vi "Compute Fit Curve v4.vi"(0 "X Array in":dbl[](array[numeric]), 1 "# Points":u32, 2 "Use Same Number of Points as Histogram":bool, 5 "Best Fit in":dbl[](array[numeric]), 7 "Y Array in":dbl[](array[numeric]), 9 "Fit Settings":T1={"Use Original Plot # Points"=TRUE, "# Fit Plot Points"=0, "Fit Method"=0, "Weighted Fit"=FALSE, "Show All Fit Components"=FALSE, "Axis Type"=0, "Show Fit Residuals"=FALSE, "Residual Type"=enum."Standard"} {"Axis Type" items=["Linear", "Logarithmic"]; "Fit Method" items=["Least Square", "Least Absolute Residual", "Bisquare"]}, 11 "Error In":errorcluster, 12 "Fit Model":T5, 13 "Fit Parameters":variant, 14 "Ramp Type":T3 items=["Linear", "Logarithmic"]) -> (3 "Array of Plots (Fit, Components, Residuals)":cluster{"X Array":dbl[], "Y Array":dbl[]}[](array[cluster]), 4 "Fitted Plot":cluster{"X Array":dbl[], "Y Array":dbl[]}, 6 "Array of Component Plots":cluster{"X Array":dbl[], "Y Array":dbl[]}[](array[cluster]), 8 "Residual Plot":cluster{"X Array":dbl[], "Y Array":dbl[]}, 10 "Residual Type":string, 15 "Error Out":errorcluster)   [LabVIEW 2019]
uses:
  Fit Models.ctl
  Calc/Ramp Type.ctl
  Fit Settings.ctl
  <vilib>/Analysis/6fits.llb/Curve Fitting Criteria.ctl
  Residual Type.ctl
  Gaussian/Gaussian Fit Results v2.ctl
  Two Connected Gaussians/Two H-Connected Gaussians Fit Parameters.ctl
  Two Connected Asymmetric Gaussians/Two H-Connected Asymmetric Gaussians Fit Parameters.ctl
  Asymmetric Gaussian/Asymmetric Gaussian Fit Results v2.ctl
  Two Connected Asymmetric Gaussians/Two T-Connected Asymmetric Gaussians Fit Parameters.ctl
  Two Connected Gaussians/Two T-Connected Gaussians Fit Parameters.ctl
  Asymmetric Lorentzian/Asymmetric Lorentzian Fit Results v2.ctl
  Gaussian-Lorentzian/Gaussian-Lorentzian Fit Results v2.ctl
  Lorentzian-Gaussian/Lorentzian-Gaussian Fit Results v2.ctl
  Lorentzian/Lorentzian Fit Results v2.ctl
  Single Exponential/Single Exponential Fit Parameters v2.ctl
  Double Exponential/Double Exponential Fit Parameters v2.ctl
  ACF-CCF/2D ACF/2D Gaussian ACF Fit Results.ctl
  ACF-CCF/2D ACF/2D Gaussian + Blinking ACF Fit Results.ctl
  ACF-CCF/2D ACF/2D Gaussian + Flow ACF Fit Results.ctl
  ACF-CCF/3D ACF/3D Gaussian ACF Fit Results.ctl
  ACF-CCF/3D ACF/3D Gaussian + Blinking ACF Fit Results.ctl
  <vilib>/Analysis/NI_AALBase.lvlib
  <vilib>/Analysis/NI_AALPro.lvlib
panel:
  out "Array of Plots (Fit, Components, Residuals)":cluster{"X Array":dbl[], "Y Array":dbl[]}[](array[cluster])
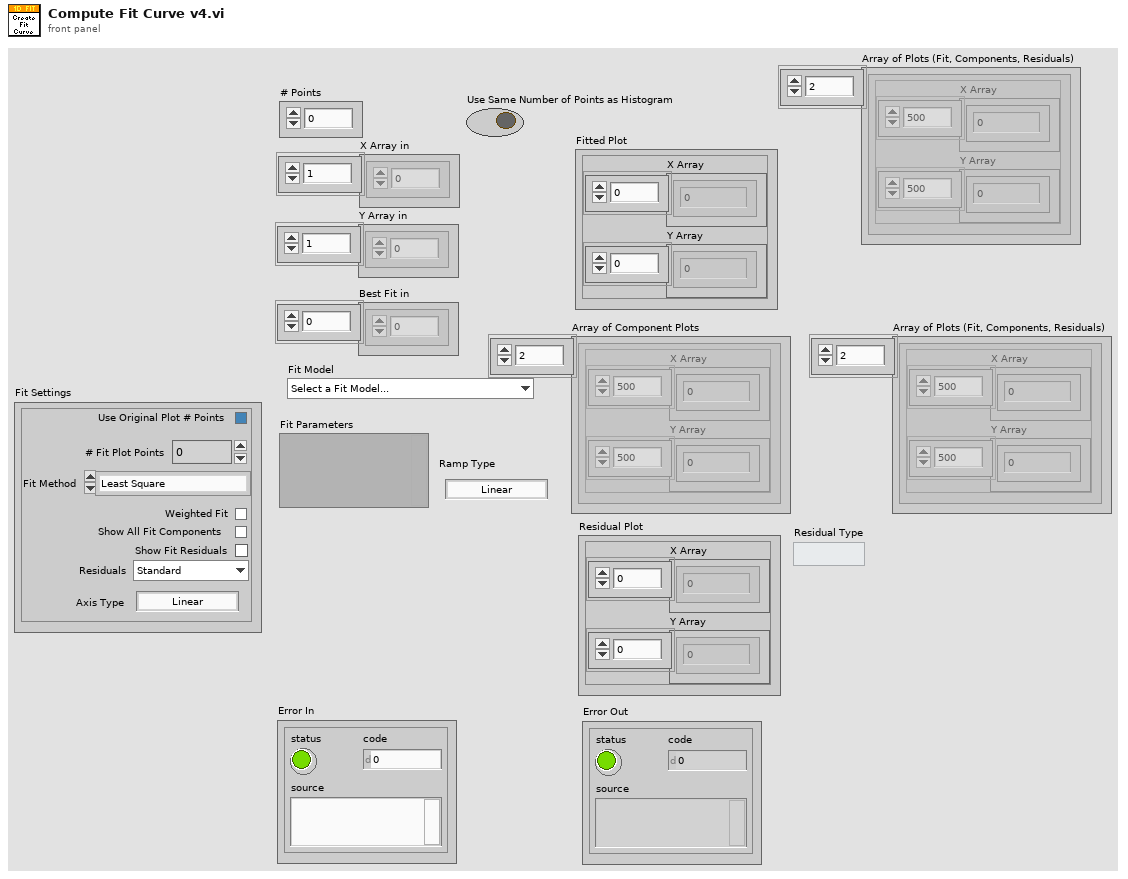
[diagram p1: front panel]
types:
  T1 = typedef "Fit Settings.ctl" = cluster{"Use Original Plot # Points":bool, "# Fit Plot Points":u32, "Fit Method":T2, "Weighted Fit":bool, "Show All Fit Components":bool, "Axis Type":T3, "Show Fit Residuals":bool, "Residual Type":T4}
  T2 = typedef "NI_AALPro.lvlib/Curve Fitting Criteria.ctl" = u16
  T3 = typedef "Ramp Type.ctl" = u16
  T4 = typedef "Residual Type.ctl" = enum16{"Standard", "Normalized", "Reduced"}
  T5 = typedef "Fit Models.ctl" = enum16{"Select a Fit Model...", "           Single Peak", "Gaussian", "Asymmetric Gaussian", "Lorentzian", "Asymmetric Lorentzian", "Gaussian/Lorentzian", "Lorentzian/Gaussian", "           Double Peak", "Two Gaussians", "Two Asymmetric Gaussians", "Two H-Connected Gaussians", "Two T-Connected Gaussians", "Two H-Connected Asymmetric Gaussians", "Two T-Connected Asymmetric Gaussians", "           Triple Peak", "Three Gaussians", "Three Asymmetric Gaussians", "              Decays", "1-Exponential", "IRF*PSED", "2-Exponentials", "               ACF", "2D Gaussian ACF", "2D Gaussian + Blinking ACF", "2D Gaussian + Flow ACF", "3D Gaussian ACF", "3D Gaussian + Blinking ACF", "             Multiplot", "2D Gaussian ACF & 2D Gaussian + Flow ACF"}
  T6 = typedef "Gaussian Fit Results v2.ctl" = cluster{"Amplitude":dbl, "Peak":dbl, "SDV":dbl, "FWHM":dbl, "Integral":dbl, "RMSE":dbl, "R^2":dbl}
  T7 = typedef "Two H-Connected Gaussians Fit Parameters.ctl" = cluster{"Gaussian Parameters":T6[], "Bridge Amplitude ":dbl}
  T8 = typedef "Two H-Connected Asymmetric Gaussians Fit Parameters.ctl" = cluster{"Asymmetric Gaussian Parameters":T9[], "Bridge Amplitude":dbl}
  T9 = typedef "Asymmetric Gaussian Fit Results v2.ctl" = cluster{"Amplitude":dbl, "Peak":dbl, "SDV-":dbl, "SDV+":dbl, "Mean":dbl, "SDV":dbl, "FWHM":dbl, "Integral":dbl, "RMSE":dbl, "R^2":dbl}
  T10 = typedef "Two T-Connected Asymmetric Gaussians Fit Parameters.ctl" = cluster{"Asymmetric Gaussian Parameters":T9[], "Bridge Amplitude":dbl, "Bridge Slope":dbl}
  T11 = typedef "Two T-Connected Gaussians Fit Parameters.ctl" = cluster{"Gaussian Parameters":T6[], "Bridge Amplitude ":dbl, "Bridge Slope":dbl}
  T12 = typedef "Asymmetric Lorentzian Fit Results v2.ctl" = cluster{"Amplitude":dbl, "Peak":dbl, "FWHM-":dbl, "FWHM+":dbl, "Integral":dbl, "RMSE":dbl, "R^2":dbl}
  T13 = typedef "Gaussian-Lorentzian Fit Results v2.ctl" = cluster{"Amplitude":dbl, "Peak":dbl, "SDV-":dbl, "FWHM+":dbl, "Mean":dbl, "FWHM":dbl, "Integral":dbl, " RMSE":dbl, "R^2":dbl}
  T14 = typedef "Lorentzian-Gaussian Fit Results v2.ctl" = cluster{"Amplitude":dbl, "Peak":dbl, "FWHM-":dbl, "SDV+":dbl, "Mean":dbl, "FWHM":dbl, "Integral":dbl, "RMSE":dbl, "R^2":dbl}
  T15 = typedef "Lorentzian Fit Results v2.ctl" = cluster{"Amplitude":dbl, "Peak":dbl, "FWHM":dbl, "Integral":dbl, "RMSE":dbl, "R^2":dbl}
  T16 = typedef "Single Exponential Fit Parameters v2.ctl" = cluster{"Amplitude":dbl, "Time Constant":dbl, "Baseline":dbl, "Mean":dbl, "SDV":dbl, "FWHM":dbl, "Integral":dbl, "MSE":dbl, "R^2":dbl}
  T17 = typedef "Double Exponential Fit Parameters v2.ctl" = cluster{"A1":dbl, "tau1":dbl, "A2":dbl, "tau2":dbl, "Baseline":dbl, "Mean":dbl, "SDV":dbl, "Integral":dbl, "MSE":dbl, "R^2":dbl}
  T18 = typedef "2D Gaussian ACF Fit Results.ctl" = cluster{"Amplitude":dbl, "Diffusion Time":dbl, "RMSE":dbl, "R^2":dbl}
  T19 = typedef "2D Gaussian + Blinking ACF Fit Results.ctl" = cluster{"Amplitude":dbl, "Diffusion Time":dbl, "Blinking Fraction":dbl, "Blinking Time Constant":dbl, "RMSE":dbl, "R^2":dbl}
  T20 = typedef "2D Gaussian + Flow ACF Fit Results.ctl" = cluster{"Amplitude":dbl, "Diffusion Time":dbl, "Translation Time":dbl, "RMSE":dbl, "R^2":dbl}
  T21 = typedef "3D Gaussian ACF Fit Results.ctl" = cluster{"Amplitude":dbl, "Diffusion Time":dbl, "Aspect Ratio":dbl, "RMSE":dbl, "R^2":dbl}
  T22 = typedef "3D Gaussian + Blinking ACF Fit Results.ctl" = cluster{"Amplitude":dbl, "Diffusion Time":dbl, "Aspect Ratio":dbl, "Blinking Fraction":dbl, "Blinking Time Constant":dbl, "RMSE":dbl, "R^2":dbl}
  T23 = typedef "IRF(X)PSED Fit Parameters.ctl" = cluster{"Offset":dbl, "Amplitudes":dbl[], "Time Constants":dbl[], "Baseline":dbl, "Lifetime":dbl, "IRF order":dbl, "Period":dbl, "SDV":dbl, "FWHM":dbl, "Integral":dbl, "MSE":dbl, "R^2":dbl}
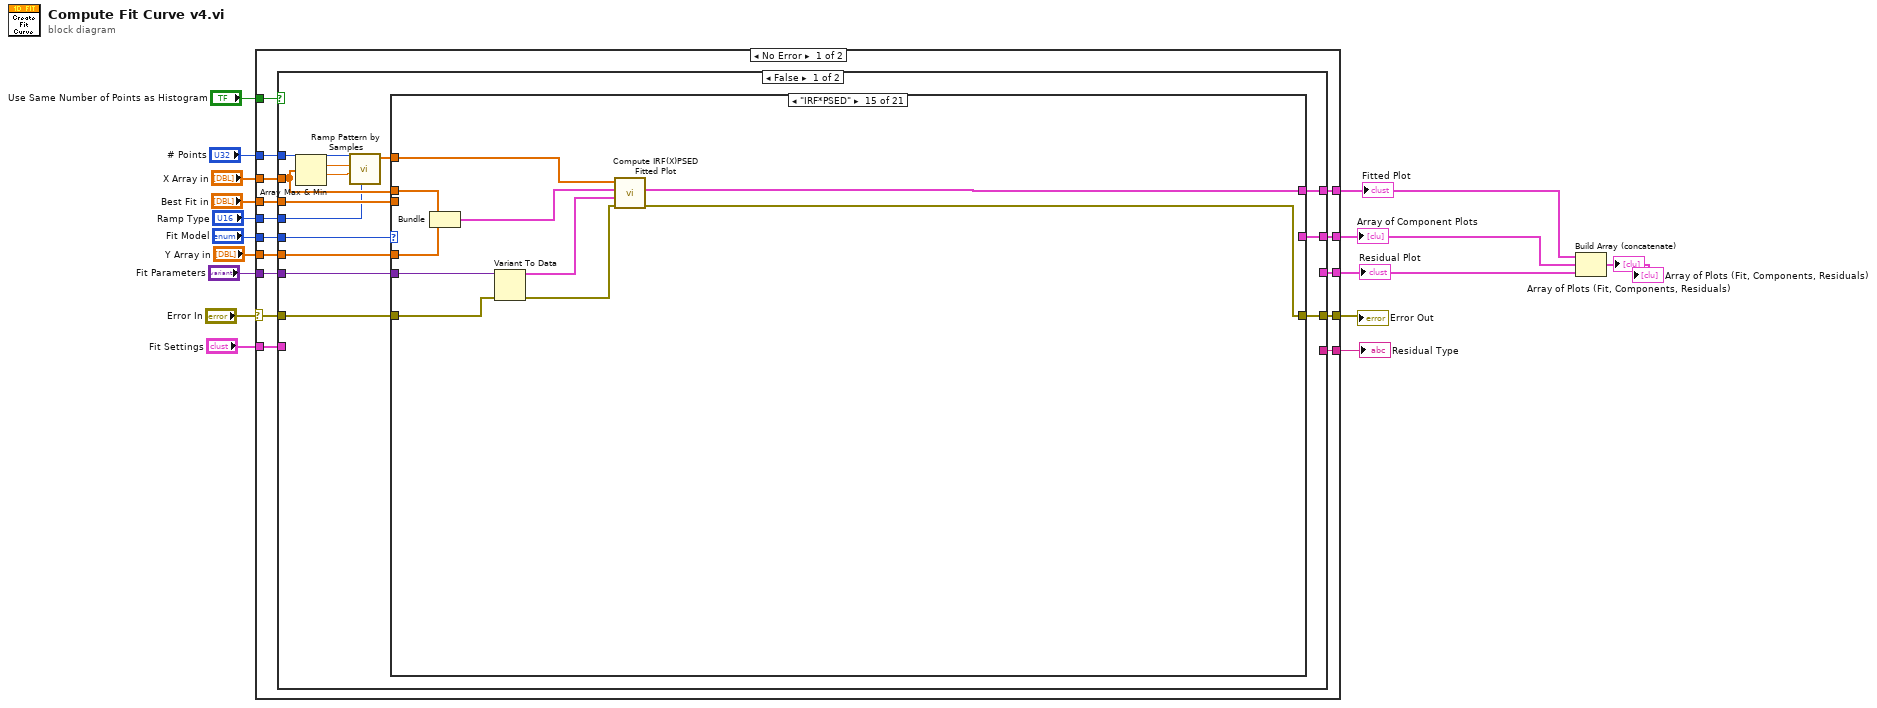
[diagram p0: block diagram]
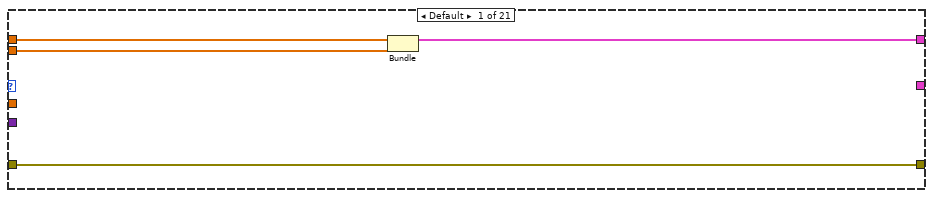
[diagram p2: hidden frame]
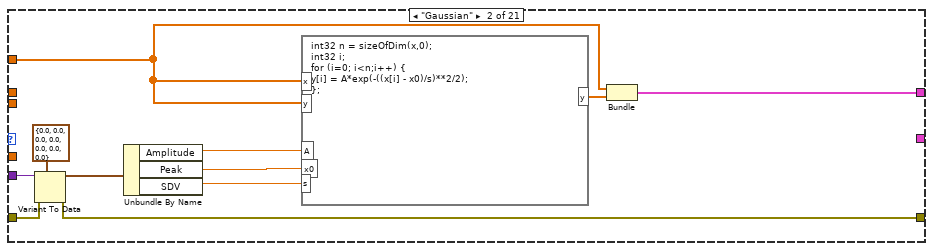
[diagram p3: hidden frame]
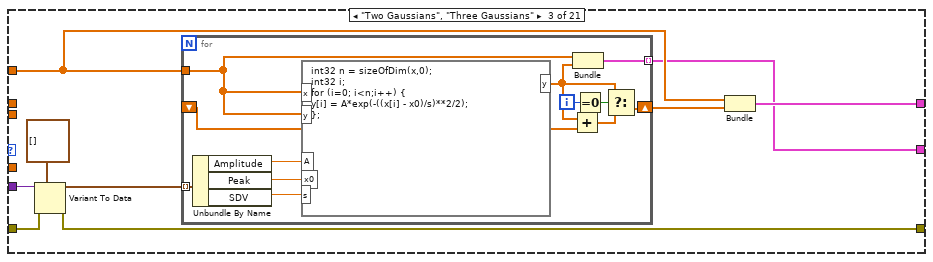
[diagram p4: hidden frame]
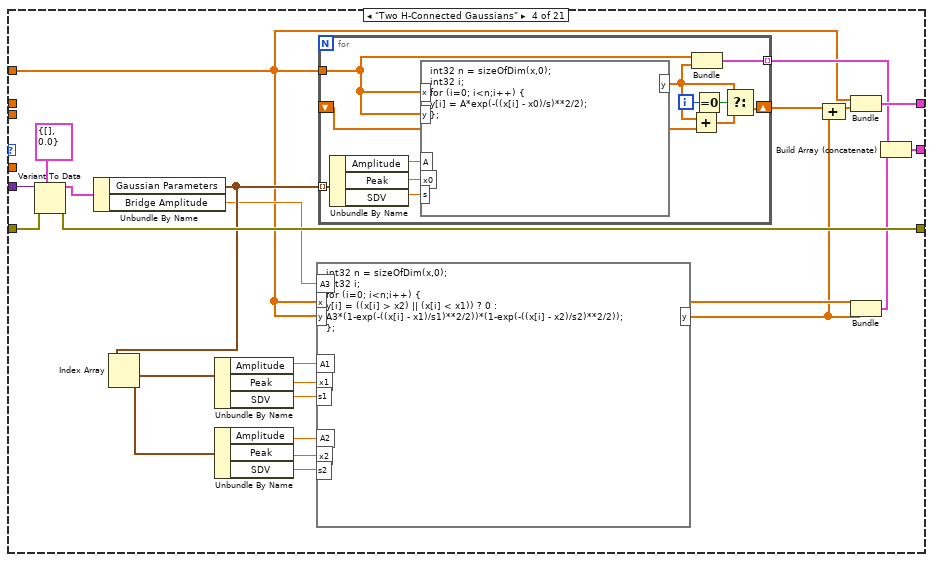
[diagram p5: hidden frame]
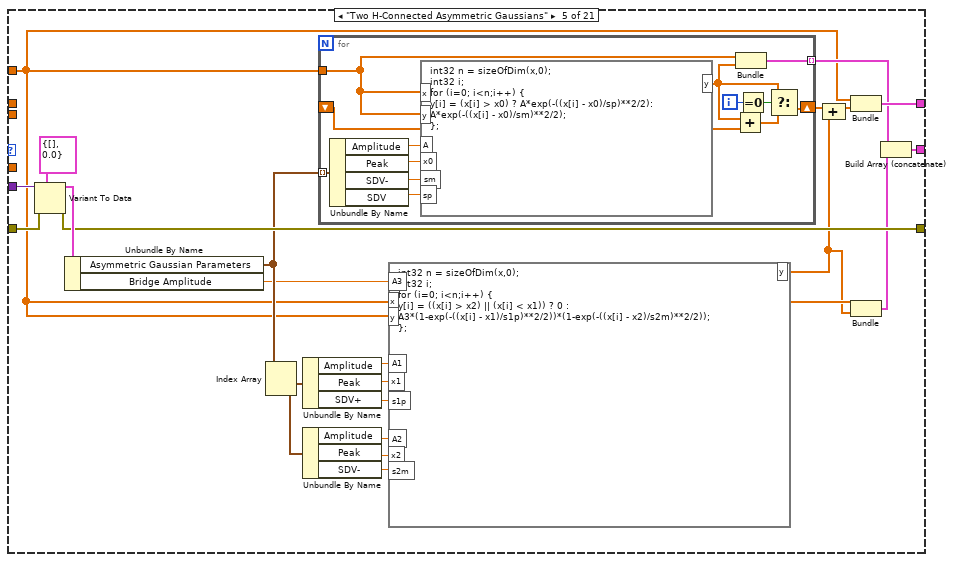
[diagram p6: hidden frame]
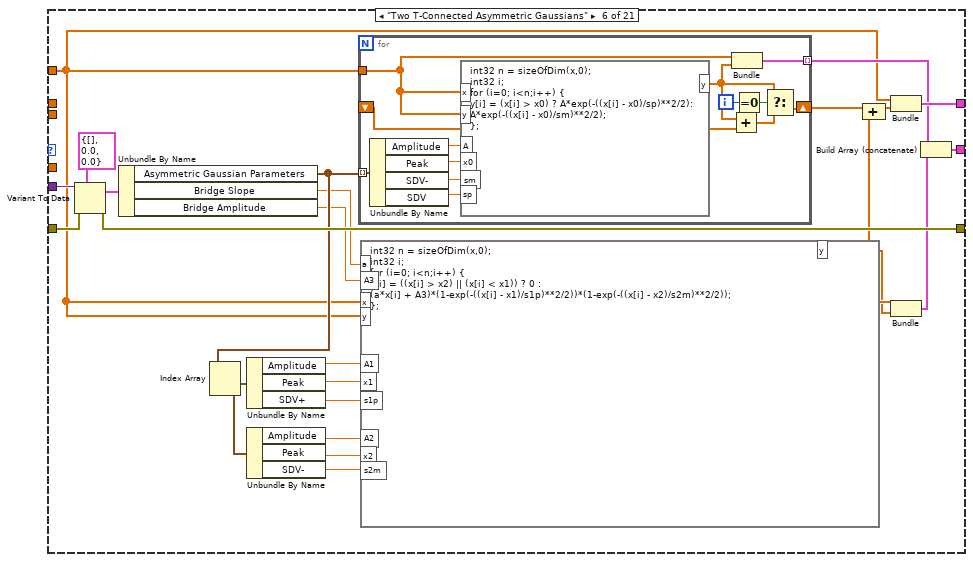
[diagram p7: hidden frame]
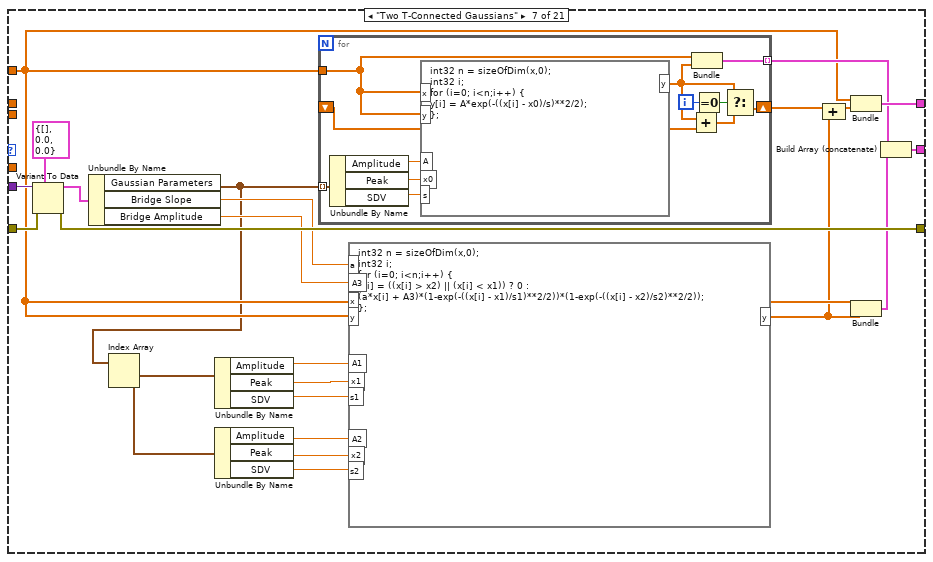
[diagram p8: hidden frame]
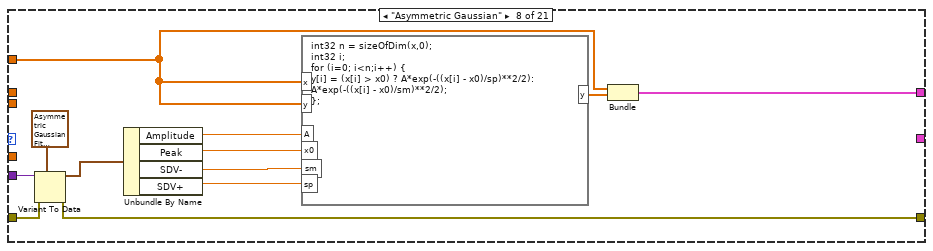
[diagram p9: hidden frame]
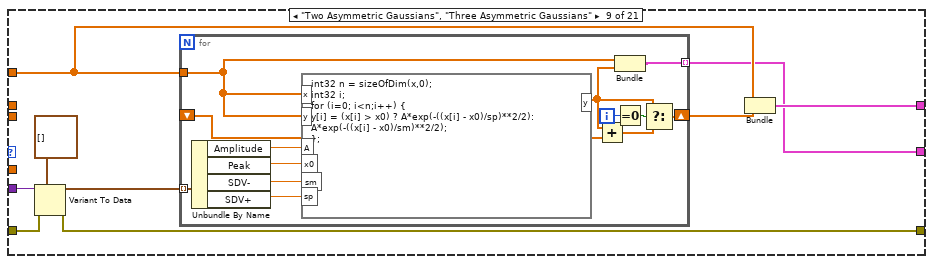
[diagram p10: hidden frame]
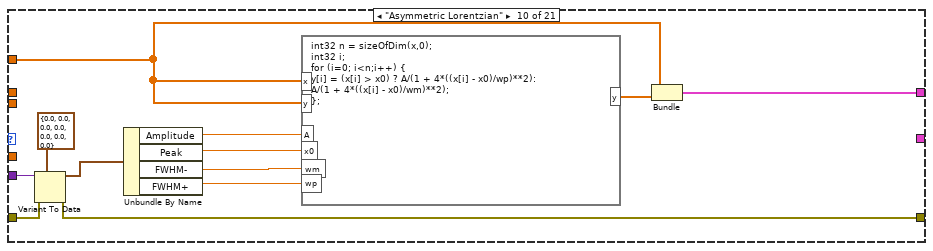
[diagram p11: hidden frame]
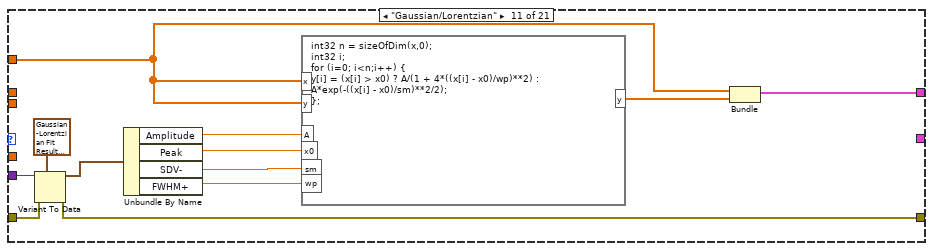
[diagram p12: hidden frame]
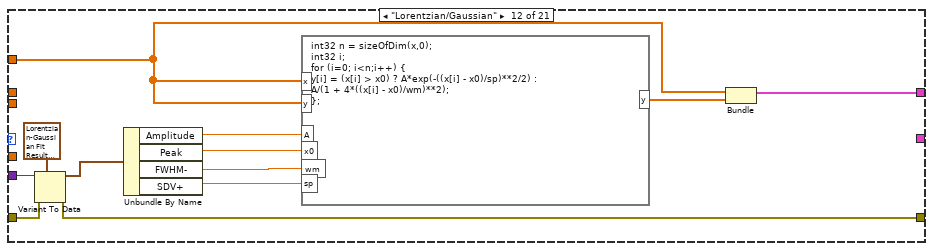
[diagram p13: hidden frame]
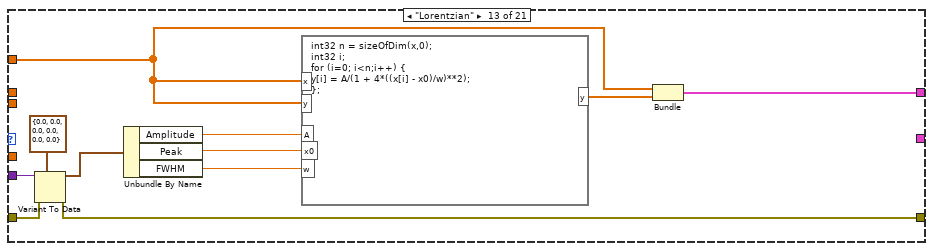
[diagram p14: hidden frame]
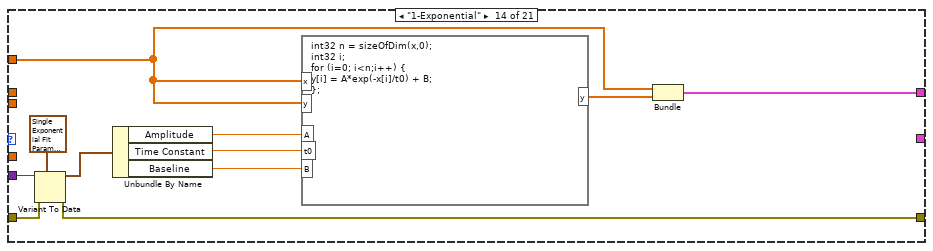
[diagram p15: hidden frame]
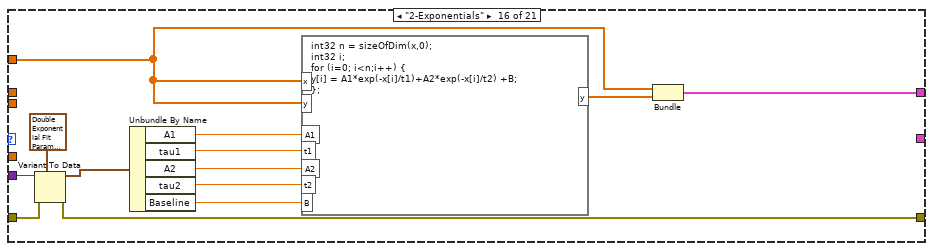
[diagram p16: hidden frame]
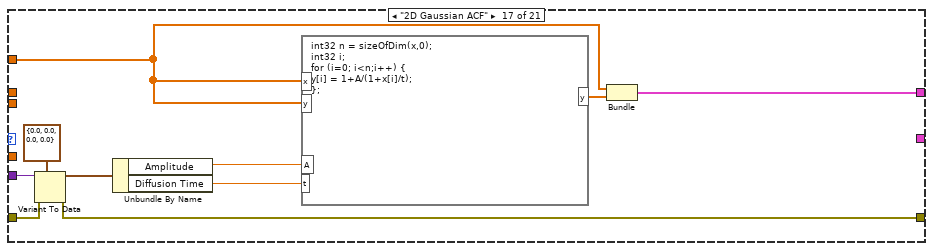
[diagram p17: hidden frame]
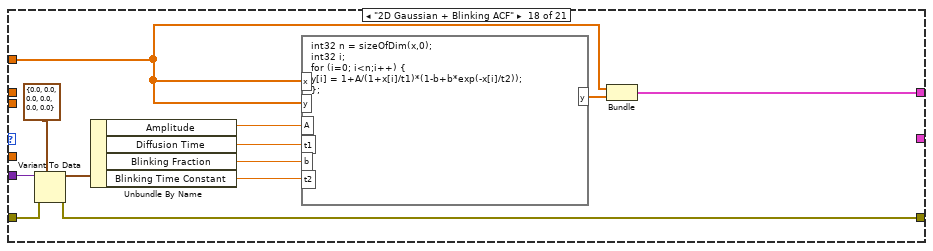
[diagram p18: hidden frame]
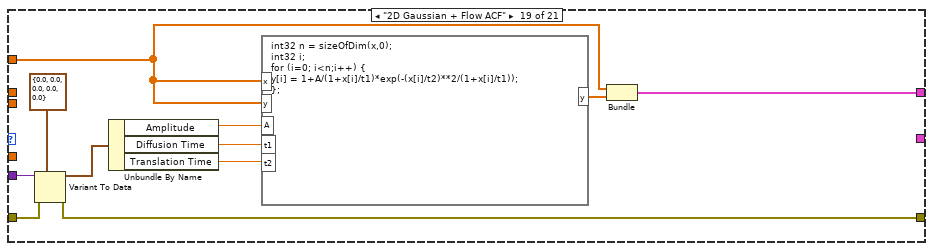
[diagram p19: hidden frame]
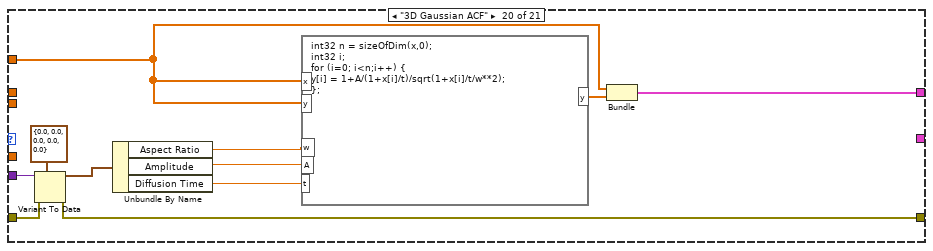
[diagram p20: hidden frame]
diagram:
  n1 = case shown="No Error" "Error In" {
    selector: "Error In" -> [w25 w434]
    tunnel: "Fit Model" -> [w31 _]
    tunnel: [w24 w434] -> w14
    tunnel: "Use Same Number of Points as Histogram" -> [w30 _]
    tunnel: "X Array in" -> [w29 w433]
    tunnel: "Best Fit in" -> [w28 w432]
    tunnel: "# Points" -> [w27 _]
    tunnel: "Fit Parameters" -> [w26 _]
    tunnel: [w22 _] -> w3
    tunnel: [w23 w431] -> w2
    tunnel: "Ramp Type" -> [w21 _]
    tunnel: [w20 _] -> w4
    tunnel: "Y Array in" -> [w19 _]
    tunnel: "Fit Settings" -> [w18 _]
    tunnel: [w17 _] -> w5
    frame No Error {
      n2 = case shown="False" w30 {
        tunnel: w31 -> [w45 _]
        tunnel: w29 -> [w38 w409]
        tunnel: w28 -> [w37 w406]
        tunnel: w27 -> [w44 _]
        tunnel: w26 -> [w40 _]
        tunnel: w25 -> [w39 w411]
        tunnel: [w36 w411] -> w24
        tunnel: [w35 w410] -> w23
        tunnel: [w34 _] -> w22
        tunnel: w21 -> [w33 _]
        tunnel: [_ w408] -> w20
        tunnel: w19 -> [w32 w407]
        tunnel: w18 -> [_ w402]
        tunnel: [_ w398] -> w17
        frame False {
          n3 = Array Max & Min(array=w38) -> (max value=w43:dbl, min value=w42:dbl)  [unwired: 2 out]
          n4 = call <vilib>:"Ramp Pattern by Samples.vi"("type"=w33, "start"=w42, "end"=w43, "samples"=w44) -> ("Ramp Pattern"=w41:dbl[])  [unwired: 6 in, 1 out]
          n5 = case shown="\"IRF*PSED\"" w45 {
            tunnel: w41 -> [_ w50 w63 w86 w122 w159 w196 w227 w240 w261 w273 w284 w296 w309 w326 w332 w341 w354 w365 w375 w389]
            tunnel: w40 -> [_ w60 w69 w104 w139 w176 w213 w237 w246 w271 w283 w295 w306 w317 w325 w340 w350 w362 w373 w384 w397]
            tunnel: w39 -> [w49 w58 w68 w103 w138 w175 w212 w236 w245 w270 w282 w294 w305 w316 w318 w339 w348 w361 w372 w382 w396]
            tunnel: w38 -> [w47 _ _ _ _ _ _ _ _ _ _ _ _ _ w324 _ _ _ _ _ _]
            tunnel: w37 -> [w48 _ _ _ _ _ _ _ _ _ _ _ _ _ _ _ _ _ _ _ _]
            tunnel: [w49 w53 w66 w101 w136 w173 w210 w230 w243 w264 w276 w288 w300 w312 w327 w335 w344 w357 w368 w378 w392] -> w36
            tunnel: [w46 w51 w62 w99 w134 w171 w208 w226 w239 w260 w272 w286 w298 w311 w321 w334 w342 w355 w366 w376 w390] -> w35
            tunnel: [_ _ w61 w93 w128 w165 w203 _ w238 _ _ _ _ _ _ _ _ _ _ _ _] -> w34
            tunnel: w32 -> [_ _ _ _ _ _ _ _ _ _ _ _ _ _ w323 _ _ _ _ _ _]
            frame Default {
              n6 = Bundle("X Array in"=w47, "Best Fit in"=w48) -> (w46:cluster{"X Array in":dbl[], "Best Fit in":dbl[]})  [unwired: 1 in]
            }
            frame "Gaussian" {
              n7 = Variant To Data(error in=w58, type=T6 {"Amplitude"=0.0, "Peak"=0.0, "SDV"=0.0, "FWHM"=0.0, "Integral"=0.0, "RMSE"=0.0, "R^2"=0.0} ("Gaussian Fit Parameters"), Variant=w60) -> (data=w57:T6, error out=w53:errorcluster)
              n8 = Unbundle By Name(w57) -> ("Amplitude"=w56:dbl, "Peak"=w55:dbl, "SDV"=w54:dbl)
              n9 = formula code="int32 n = sizeOfDim(x,0);\nint32 i;\nfor (i=0; i<n;i++) {\ny[i] = A*exp(-((x[i] - x0)/s)**2/2);\n};"("A"=w56, "x0"=w55, "s"=w54, "x"=w50, "y"=w50) -> ("y"=w52:dbl[])
              n10 = Bundle("Ramp Pattern"=w50, "y"=w52) -> (w51:cluster{"Ramp Pattern":dbl[], "y":dbl[]})  [unwired: 1 in]
            }
            frame "Two Gaussians", "Three Gaussians" {
              n11 = Variant To Data(error in=w68, type=T6[] [] ("Two Gaussians Fit Parameters"), Variant=w69) -> (data=w67:T6[], error out=w66:errorcluster)
              n12 = for {
                tunnel: w67 -> [w81] mode=indexing
                tunnel: w63 -> [w71]
                shift-right: [w74] -> w64
                shift-left: _ -> [w75]
                tunnel: [w70] -> w61 mode=indexing
                i -> [w77]
                n13 = Unbundle By Name(w81) -> ("Amplitude"=w80:dbl, "Peak"=w79:dbl, "SDV"=w78:dbl)
                n14 = formula code="int32 n = sizeOfDim(x,0);\nint32 i;\nfor (i=0; i<n;i++) {\ny[i] = A*exp(-((x[i] - x0)/s)**2/2);\n};"("A"=w80, "x0"=w79, "s"=w78, "x"=w71, "y"=w71) -> ("y"=w72:dbl[])
                n15 = Add(x=w72, y=w75) -> (x+y=w73:dbl[])
                n16 = Bundle("Ramp Pattern"=w71, "y"=w72) -> (w70:cluster{"Ramp Pattern":dbl[], "y":dbl[]})  [unwired: 1 in]
                n17 = Equal To 0?(x=w77) -> (x = 0?=w76:bool)
                n18 = Select(t=w72, s=w76, f=w73) -> (s? t:f=w74:dbl[])
              }
              n19 = Bundle("Ramp Pattern"=w63, "y"=w64) -> (w62:cluster{"Ramp Pattern":dbl[], "y":dbl[]})  [unwired: 1 in]
            }
            frame "Two H-Connected Gaussians" {
              n20 = Variant To Data(error in=w103, type=T7 {"Gaussian Parameters"=[], "Bridge Amplitude "=0.0} ("Bridged Gaussians Parameters"), Variant=w104) -> (data=w102:T7, error out=w101:errorcluster)
              n21 = Unbundle By Name(w102) -> ("Gaussian Parameters"=w97:T6[], "Bridge Amplitude"=w94:dbl)
              n22 = Index Array(array=w97) -> (element #1=w96:T6, element #2=w95:T6)  [unwired: 2 in]
              n23 = Unbundle By Name(w96) -> ("Amplitude"=w92:dbl, "Peak"=w91:dbl, "SDV"=w90:dbl)
              n24 = Unbundle By Name(w95) -> ("Amplitude"=w87:dbl, "Peak"=w88:dbl, "SDV"=w89:dbl)
              n25 = formula code="int32 n = sizeOfDim(x,0);\nint32 i;\nfor (i=0; i<n;i++) {\ny[i] = ((x[i] > x2) || (x[i] < x1)) ? 0 : \nA3*(1-exp(-((x[i] - x1)/s1)**2/2))*(1-exp(-((x[i] - x2)/s2)**2/2));\n};"("A1"=w92, "x1"=w91, "s1"=w90, "x"=w86, "y"=w86, "A2"=w87, "x2"=w88, "s2"=w89, "A3"=w94) -> ("y"=w83:dbl[])
              n26 = for {
                tunnel: w97 -> [w116] mode=indexing
                tunnel: w86 -> [w106]
                shift-right: [w109] -> w100
                shift-left: _ -> [w110]
                tunnel: [w105] -> w98 mode=indexing
                i -> [w112]
                n27 = Unbundle By Name(w116) -> ("Amplitude"=w115:dbl, "Peak"=w114:dbl, "SDV"=w113:dbl)
                n28 = formula code="int32 n = sizeOfDim(x,0);\nint32 i;\nfor (i=0; i<n;i++) {\ny[i] = A*exp(-((x[i] - x0)/s)**2/2);\n};"("A"=w115, "x0"=w114, "s"=w113, "x"=w106, "y"=w106) -> ("y"=w107:dbl[])
                n29 = Add(x=w107, y=w110) -> (x+y=w108:dbl[])
                n30 = Bundle("Ramp Pattern"=w106, "y"=w107) -> (w105:cluster{"Ramp Pattern":dbl[], "y":dbl[]})  [unwired: 1 in]
                n31 = Equal To 0?(x=w112) -> (x = 0?=w111:bool)
                n32 = Select(t=w107, s=w111, f=w108) -> (s? t:f=w109:dbl[])
              }
              n33 = Compound Arithmetic op=ADD(w100, w83) -> (w84:dbl[])
              n34 = Bundle("Ramp Pattern"=w86, w84) -> (w99:cluster{"Ramp Pattern":dbl[], dbl[]})  [unwired: 1 in]
              n35 = Bundle("Ramp Pattern"=w86, "y"=w83) -> (w85:cluster{"Ramp Pattern":dbl[], "y":dbl[]})  [unwired: 1 in]
              n36 = Build Array (concatenate)(w98, w85) -> (w93:cluster{"Ramp Pattern":dbl[], "y":dbl[]}[])
            }
            frame "Two H-Connected Asymmetric Gaussians" {
              n37 = Variant To Data(error in=w138, type=T8 {"Asymmetric Gaussian Parameters"=[], "Bridge Amplitude"=0.0} ("output cluster"), Variant=w139) -> (data=w137:T8, error out=w136:errorcluster)
              n38 = Unbundle By Name(w137) -> ("Asymmetric Gaussian Parameters"=w132:T9[], "Bridge Amplitude"=w129:dbl)
              n39 = Index Array(array=w132) -> (element #1=w131:T9, element #2=w130:T9)  [unwired: 2 in]
              n40 = Unbundle By Name(w131) -> ("Amplitude"=w127:dbl, "Peak"=w126:dbl, "SDV+"=w118:dbl)
              n41 = Unbundle By Name(w130) -> ("Amplitude"=w123:dbl, "Peak"=w124:dbl, "SDV-"=w125:dbl)
              n42 = for {
                tunnel: w132 -> [w152] mode=indexing
                tunnel: w122 -> [w141]
                shift-right: [w144] -> w135
                shift-left: _ -> [w145]
                tunnel: [w140] -> w133 mode=indexing
                i -> [w147]
                n43 = Unbundle By Name(w152) -> ("Amplitude"=w151:dbl, "Peak"=w150:dbl, "SDV-"=w149:dbl, "SDV"=w148:dbl)
                n44 = formula code="int32 n = sizeOfDim(x,0);\nint32 i;\nfor (i=0; i<n;i++) {\ny[i] = (x[i] > x0) ? A*exp(-((x[i] - x0)/sp)**2/2):\nA*exp(-((x[i] - x0)/sm)**2/2);\n};"("A"=w151, "x0"=w150, "sm"=w149, "sp"=w148, "x"=w141, "y"=w141) -> ("y"=w142:dbl[])
                n45 = Add(x=w142, y=w145) -> (x+y=w143:dbl[])
                n46 = Bundle("Ramp Pattern"=w141, "y"=w142) -> (w140:cluster{"Ramp Pattern":dbl[], "y":dbl[]})  [unwired: 1 in]
                n47 = Equal To 0?(x=w147) -> (x = 0?=w146:bool)
                n48 = Select(t=w142, s=w146, f=w143) -> (s? t:f=w144:dbl[])
              }
              n49 = formula code="int32 n = sizeOfDim(x,0);\nint32 i;\nfor (i=0; i<n;i++) {\ny[i] = ((x[i] > x2) || (x[i] < x1)) ? 0 : \nA3*(1-exp(-((x[i] - x1)/s1p)**2/2))*(1-exp(-((x[i] - x2)/s2m)**2/2));\n};"("A1"=w127, "x1"=w126, "x"=w122, "y"=w122, "A2"=w123, "x2"=w124, "s2m"=w125, "A3"=w129, "s1p"=w118) -> ("y"=w119:dbl[])
              n50 = Compound Arithmetic op=ADD(w135, w119) -> (w120:dbl[])
              n51 = Bundle("Ramp Pattern"=w122, w120) -> (w134:cluster{"Ramp Pattern":dbl[], dbl[]})  [unwired: 1 in]
              n52 = Bundle("Ramp Pattern"=w122, "y"=w119) -> (w121:cluster{"Ramp Pattern":dbl[], "y":dbl[]})  [unwired: 1 in]
              n53 = Build Array (concatenate)(w133, w121) -> (w128:cluster{"Ramp Pattern":dbl[], "y":dbl[]}[])
            }
            frame "Two T-Connected Asymmetric Gaussians" {
              n54 = Variant To Data(error in=w175, type=T10 {"Asymmetric Gaussian Parameters"=[], "Bridge Amplitude"=0.0, "Bridge Slope"=0.0} ("Two T-Connected Asymmetric Gaussian Parameters"), Variant=w176) -> (data=w174:T10, error out=w173:errorcluster)
              n55 = Unbundle By Name(w174) -> ("Asymmetric Gaussian Parameters"=w169:T9[], "Bridge Slope"=w166:dbl, "Bridge Amplitude"=w154:dbl)
              n56 = Index Array(array=w169) -> (element #1=w168:T9, element #2=w167:T9)  [unwired: 2 in]
              n57 = Unbundle By Name(w168) -> ("Amplitude"=w164:dbl, "Peak"=w163:dbl, "SDV+"=w155:dbl)
              n58 = Unbundle By Name(w167) -> ("Amplitude"=w160:dbl, "Peak"=w161:dbl, "SDV-"=w162:dbl)
              n59 = for {
                tunnel: w169 -> [w189] mode=indexing
                tunnel: w159 -> [w178]
                shift-right: [w181] -> w172
                shift-left: _ -> [w182]
                tunnel: [w177] -> w170 mode=indexing
                i -> [w184]
                n60 = Unbundle By Name(w189) -> ("Amplitude"=w188:dbl, "Peak"=w187:dbl, "SDV-"=w186:dbl, "SDV"=w185:dbl)
                n61 = formula code="int32 n = sizeOfDim(x,0);\nint32 i;\nfor (i=0; i<n;i++) {\ny[i] = (x[i] > x0) ? A*exp(-((x[i] - x0)/sp)**2/2):\nA*exp(-((x[i] - x0)/sm)**2/2);\n};"("A"=w188, "x0"=w187, "sm"=w186, "sp"=w185, "x"=w178, "y"=w178) -> ("y"=w179:dbl[])
                n62 = Add(x=w179, y=w182) -> (x+y=w180:dbl[])
                n63 = Bundle("Ramp Pattern"=w178, "y"=w179) -> (w177:cluster{"Ramp Pattern":dbl[], "y":dbl[]})  [unwired: 1 in]
                n64 = Equal To 0?(x=w184) -> (x = 0?=w183:bool)
                n65 = Select(t=w179, s=w183, f=w180) -> (s? t:f=w181:dbl[])
              }
              n66 = formula code="int32 n = sizeOfDim(x,0);\nint32 i;\nfor (i=0; i<n;i++) {\ny[i] = ((x[i] > x2) || (x[i] < x1)) ? 0 : \n(a*x[i] + A3)*(1-exp(-((x[i] - x1)/s1p)**2/2))*(1-exp(-((x[i] - x2)/s2m)**2/2));\n};"("A1"=w164, "x1"=w163, "x"=w159, "y"=w159, "A2"=w160, "x2"=w161, "s2m"=w162, "a"=w166, "s1p"=w155, "A3"=w154) -> ("y"=w156:dbl[])
              n67 = Compound Arithmetic op=ADD(w172, w156) -> (w157:dbl[])
              n68 = Bundle("Ramp Pattern"=w159, w157) -> (w171:cluster{"Ramp Pattern":dbl[], dbl[]})  [unwired: 1 in]
              n69 = Bundle("Ramp Pattern"=w159, "y"=w156) -> (w158:cluster{"Ramp Pattern":dbl[], "y":dbl[]})  [unwired: 1 in]
              n70 = Build Array (concatenate)(w170, w158) -> (w165:cluster{"Ramp Pattern":dbl[], "y":dbl[]}[])
            }
            frame "Two T-Connected Gaussians" {
              n71 = Variant To Data(error in=w212, type=T11 {"Gaussian Parameters"=[], "Bridge Amplitude "=0.0, "Bridge Slope"=0.0} ("Bridged Gaussians Parameters"), Variant=w213) -> (data=w211:T11, error out=w210:errorcluster)
              n72 = Unbundle By Name(w211) -> ("Gaussian Parameters"=w190:T6[], "Bridge Slope"=w204:dbl, "Bridge Amplitude"=w192:dbl)
              n73 = Index Array(array=w190) -> (element #1=w206:T6, element #2=w205:T6)  [unwired: 2 in]
              n74 = Unbundle By Name(w206) -> ("Amplitude"=w202:dbl, "Peak"=w201:dbl, "SDV"=w200:dbl)
              n75 = Unbundle By Name(w205) -> ("Amplitude"=w197:dbl, "Peak"=w198:dbl, "SDV"=w199:dbl)
              n76 = for {
                tunnel: w190 -> [w225] mode=indexing
                tunnel: w196 -> [w215]
                shift-right: [w218] -> w209
                shift-left: _ -> [w219]
                tunnel: [w214] -> w207 mode=indexing
                i -> [w221]
                n77 = Unbundle By Name(w225) -> ("Amplitude"=w224:dbl, "Peak"=w223:dbl, "SDV"=w222:dbl)
                n78 = formula code="int32 n = sizeOfDim(x,0);\nint32 i;\nfor (i=0; i<n;i++) {\ny[i] = A*exp(-((x[i] - x0)/s)**2/2);\n};"("A"=w224, "x0"=w223, "s"=w222, "x"=w215, "y"=w215) -> ("y"=w216:dbl[])
                n79 = Add(x=w216, y=w219) -> (x+y=w217:dbl[])
                n80 = Bundle("Ramp Pattern"=w215, "y"=w216) -> (w214:cluster{"Ramp Pattern":dbl[], "y":dbl[]})  [unwired: 1 in]
                n81 = Equal To 0?(x=w221) -> (x = 0?=w220:bool)
                n82 = Select(t=w216, s=w220, f=w217) -> (s? t:f=w218:dbl[])
              }
              n83 = formula code="int32 n = sizeOfDim(x,0);\nint32 i;\nfor (i=0; i<n;i++) {\ny[i] = ((x[i] > x2) || (x[i] < x1)) ? 0 : \n(a*x[i] + A3)*(1-exp(-((x[i] - x1)/s1)**2/2))*(1-exp(-((x[i] - x2)/s2)**2/2));\n};"("A1"=w202, "x1"=w201, "s1"=w200, "x"=w196, "y"=w196, "A2"=w197, "x2"=w198, "s2"=w199, "a"=w204, "A3"=w192) -> ("y"=w193:dbl[])
              n84 = Compound Arithmetic op=ADD(w209, w193) -> (w194:dbl[])
              n85 = Bundle("Ramp Pattern"=w196, w194) -> (w208:cluster{"Ramp Pattern":dbl[], dbl[]})  [unwired: 1 in]
              n86 = Bundle("Ramp Pattern"=w196, "y"=w193) -> (w195:cluster{"Ramp Pattern":dbl[], "y":dbl[]})  [unwired: 1 in]
              n87 = Build Array (concatenate)(w207, w195) -> (w203:cluster{"Ramp Pattern":dbl[], "y":dbl[]}[])
            }
            frame "Asymmetric Gaussian" {
              n88 = Variant To Data(error in=w236, type=T9 {"Amplitude"=0.0, "Peak"=0.0, "SDV-"=0.0, "SDV+"=0.0, "Mean"=0.0, "SDV"=0.0, "FWHM"=0.0, "Integral"=0.0, "RMSE"=0.0, "R^2"=0.0} ("Asymmetric Gaussian Fit Parameters"), Variant=w237) -> (data=w235:T9, error out=w230:errorcluster)
              n89 = Unbundle By Name(w235) -> ("Amplitude"=w234:dbl, "Peak"=w233:dbl, "SDV-"=w232:dbl, "SDV+"=w231:dbl)
              n90 = formula code="int32 n = sizeOfDim(x,0);\nint32 i;\nfor (i=0; i<n;i++) {\ny[i] = (x[i] > x0) ? A*exp(-((x[i] - x0)/sp)**2/2):\nA*exp(-((x[i] - x0)/sm)**2/2);\n};"("A"=w234, "x0"=w233, "sm"=w232, "sp"=w231, "x"=w227, "y"=w227) -> ("y"=w228:dbl[])
              n91 = Bundle("Ramp Pattern"=w227, "y"=w228) -> (w226:cluster{"Ramp Pattern":dbl[], "y":dbl[]})  [unwired: 1 in]
            }
            frame "Two Asymmetric Gaussians", "Three Asymmetric Gaussians" {
              n92 = Variant To Data(error in=w245, type=T9[] [] ("Two Asymmetric Gaussians Fit Parameters"), Variant=w246) -> (data=w244:T9[], error out=w243:errorcluster)
              n93 = for {
                tunnel: w244 -> [w259] mode=indexing
                tunnel: w240 -> [w248]
                shift-right: [w252] -> w241
                shift-left: _ -> [w251]
                tunnel: [w247] -> w238 mode=indexing
                i -> [w253]
                n94 = Unbundle By Name(w259) -> ("Amplitude"=w258:dbl, "Peak"=w257:dbl, "SDV-"=w256:dbl, "SDV+"=w255:dbl)
                n95 = formula code="int32 n = sizeOfDim(x,0);\nint32 i;\nfor (i=0; i<n;i++) {\ny[i] = (x[i] > x0) ? A*exp(-((x[i] - x0)/sp)**2/2):\nA*exp(-((x[i] - x0)/sm)**2/2);\n};"("A"=w258, "x0"=w257, "sm"=w256, "sp"=w255, "x"=w248, "y"=w248) -> ("y"=w249:dbl[])
                n96 = Add(x=w249, y=w251) -> (x+y=w250:dbl[])
                n97 = Bundle("Ramp Pattern"=w248, "y"=w249) -> (w247:cluster{"Ramp Pattern":dbl[], "y":dbl[]})  [unwired: 1 in]
                n98 = Equal To 0?(x=w253) -> (x = 0?=w254:bool)
                n99 = Select(t=w249, s=w254, f=w250) -> (s? t:f=w252:dbl[])
              }
              n100 = Bundle("Ramp Pattern"=w240, "y"=w241) -> (w239:cluster{"Ramp Pattern":dbl[], "y":dbl[]})  [unwired: 1 in]
            }
            frame "Asymmetric Lorentzian" {
              n101 = Variant To Data(error in=w270, type=T12 {"Amplitude"=0.0, "Peak"=0.0, "FWHM-"=0.0, "FWHM+"=0.0, "Integral"=0.0, "RMSE"=0.0, "R^2"=0.0} ("Asymmetric Lorentz Fit Parameters"), Variant=w271) -> (data=w269:T12, error out=w264:errorcluster)
              n102 = Unbundle By Name(w269) -> ("Amplitude"=w268:dbl, "Peak"=w267:dbl, "FWHM-"=w266:dbl, "FWHM+"=w265:dbl)
              n103 = formula code="int32 n = sizeOfDim(x,0);\nint32 i;\nfor (i=0; i<n;i++) {\ny[i] = (x[i] > x0) ? A/(1 + 4*((x[i] - x0)/wp)**2):\nA/(1 + 4*((x[i] - x0)/wm)**2);\n};"("A"=w268, "x0"=w267, "wm"=w266, "wp"=w265, "x"=w261, "y"=w261) -> ("y"=w262:dbl[])
              n104 = Bundle("Ramp Pattern"=w261, "y"=w262) -> (w260:cluster{"Ramp Pattern":dbl[], "y":dbl[]})  [unwired: 1 in]
            }
            frame "Gaussian/Lorentzian" {
              n105 = Variant To Data(error in=w282, type=T13 {"Amplitude"=0.0, "Peak"=0.0, "SDV-"=0.0, "FWHM+"=0.0, "Mean"=0.0, "FWHM"=0.0, "Integral"=0.0, " RMSE"=0.0, "R^2"=0.0} ("Gaussian/Lorentzian Fit Parameters"), Variant=w283) -> (data=w281:T13, error out=w276:errorcluster)
              n106 = Unbundle By Name(w281) -> ("Amplitude"=w280:dbl, "Peak"=w279:dbl, "SDV-"=w278:dbl, "FWHM+"=w277:dbl)
              n107 = formula code="int32 n = sizeOfDim(x,0);\nint32 i;\nfor (i=0; i<n;i++) {\ny[i] = (x[i] > x0) ? A/(1 + 4*((x[i] - x0)/wp)**2) :\nA*exp(-((x[i] - x0)/sm)**2/2);\n};"("A"=w280, "x0"=w279, "sm"=w278, "wp"=w277, "x"=w273, "y"=w273) -> ("y"=w274:dbl[])
              n108 = Bundle("Ramp Pattern"=w273, "y"=w274) -> (w272:cluster{"Ramp Pattern":dbl[], "y":dbl[]})  [unwired: 1 in]
            }
            frame "Lorentzian/Gaussian" {
              n109 = Variant To Data(error in=w294, type=T14 {"Amplitude"=0.0, "Peak"=0.0, "FWHM-"=0.0, "SDV+"=0.0, "Mean"=0.0, "FWHM"=0.0, "Integral"=0.0, "RMSE"=0.0, "R^2"=0.0} ("Lorentzian/Gaussian Fit Parameters"), Variant=w295) -> (data=w293:T14, error out=w288:errorcluster)
              n110 = Unbundle By Name(w293) -> ("Amplitude"=w292:dbl, "Peak"=w291:dbl, "FWHM-"=w290:dbl, "SDV+"=w289:dbl)
              n111 = formula code="int32 n = sizeOfDim(x,0);\nint32 i;\nfor (i=0; i<n;i++) {\ny[i] = (x[i] > x0) ? A*exp(-((x[i] - x0)/sp)**2/2) :\nA/(1 + 4*((x[i] - x0)/wm)**2);\n};"("A"=w292, "x0"=w291, "wm"=w290, "sp"=w289, "x"=w284, "y"=w284) -> ("y"=w285:dbl[])
              n112 = Bundle("Ramp Pattern"=w284, "y"=w285) -> (w286:cluster{"Ramp Pattern":dbl[], "y":dbl[]})  [unwired: 1 in]
            }
            frame "Lorentzian" {
              n113 = Variant To Data(error in=w305, type=T15 {"Amplitude"=0.0, "Peak"=0.0, "FWHM"=0.0, "Integral"=0.0, "RMSE"=0.0, "R^2"=0.0} ("Lorentz Fit Parameters"), Variant=w306) -> (data=w304:T15, error out=w300:errorcluster)
              n114 = Unbundle By Name(w304) -> ("Amplitude"=w303:dbl, "Peak"=w302:dbl, "FWHM"=w301:dbl)
              n115 = formula code="int32 n = sizeOfDim(x,0);\nint32 i;\nfor (i=0; i<n;i++) {\ny[i] = A/(1 + 4*((x[i] - x0)/w)**2);\n};"("A"=w303, "x0"=w302, "w"=w301, "x"=w296, "y"=w296) -> ("y"=w297:dbl[])
              n116 = Bundle("Ramp Pattern"=w296, "y"=w297) -> (w298:cluster{"Ramp Pattern":dbl[], "y":dbl[]})  [unwired: 1 in]
            }
            frame "1-Exponential" {
              n117 = Variant To Data(error in=w316, type=T16 {"Amplitude"=0.0, "Time Constant"=0.0, "Baseline"=0.0, "Mean"=0.0, "SDV"=0.0, "FWHM"=0.0, "Integral"=0.0, "MSE"=0.0, "R^2"=0.0} ("Single Exponential Fit Parameters"), Variant=w317) -> (data=w315:T16, error out=w312:errorcluster)
              n118 = Unbundle By Name(w315) -> ("Amplitude"=w314:dbl, "Time Constant"=w313:dbl, "Baseline"=w307:dbl)
              n119 = formula code="int32 n = sizeOfDim(x,0);\nint32 i;\nfor (i=0; i<n;i++) {\ny[i] = A*exp(-x[i]/t0) + B;\n};"("A"=w314, "t0"=w313, "x"=w309, "y"=w309, "B"=w307) -> ("y"=w310:dbl[])
              n120 = Bundle("Ramp Pattern"=w309, "y"=w310) -> (w311:cluster{"Ramp Pattern":dbl[], "y":dbl[]})  [unwired: 1 in]
            }
            frame "IRF*PSED" {
              n121 = Bundle("X Array in"=w324, "Y Array in"=w323) -> (w322:cluster{"X Array in":dbl[], "Y Array in":dbl[]})  [unwired: 1 in]
              n122 = Variant To Data(error in=w318, Variant=w325) -> (data=w320:T23, error out=w319:errorcluster)  [unwired: 1 in]
              n123 = call "Compute IRF(X)PSED Fitted Plot.vi"("error in (no error)"=w319, "IRF*PSED Fit Parameters"=w320, "Original Plot"=w322, "Ramp Pattern"=w326) -> ("error out"=w327:errorcluster, "Fitted Plot"=w321:cluster{"X Array":dbl[], "Y Array":dbl[]})  [unwired: 6 in]
            }
            frame "2-Exponentials" {
              n124 = Variant To Data(error in=w339, type=T17 {"A1"=0.0, "tau1"=0.0, "A2"=0.0, "tau2"=0.0, "Baseline"=0.0, "Mean"=0.0, "SDV"=0.0, "Integral"=0.0, "MSE"=0.0, "R^2"=0.0} ("Double Exponential Fit Parameters"), Variant=w340) -> (data=w338:T17, error out=w335:errorcluster)
              n125 = Unbundle By Name(w338) -> ("A1"=w337:dbl, "tau1"=w336:dbl, "A2"=w330:dbl, "tau2"=w329:dbl, "Baseline"=w328:dbl)
              n126 = formula code="int32 n = sizeOfDim(x,0);\nint32 i;\nfor (i=0; i<n;i++) {\ny[i] = A1*exp(-x[i]/t1)+A2*exp(-x[i]/t2) +B;\n};"("A1"=w337, "t1"=w336, "x"=w332, "y"=w332, "A2"=w330, "t2"=w329, "B"=w328) -> ("y"=w333:dbl[])
              n127 = Bundle("Ramp Pattern"=w332, "y"=w333) -> (w334:cluster{"Ramp Pattern":dbl[], "y":dbl[]})  [unwired: 1 in]
            }
            frame "2D Gaussian ACF" {
              n128 = Variant To Data(error in=w348, type=T18 {"Amplitude"=0.0, "Diffusion Time"=0.0, "RMSE"=0.0, "R^2"=0.0} ("2D ACF Fit Parameters"), Variant=w350) -> (data=w347:T18, error out=w344:errorcluster)
              n129 = Unbundle By Name(w347) -> ("Amplitude"=w346:dbl, "Diffusion Time"=w345:dbl)
              n130 = formula code="int32 n = sizeOfDim(x,0);\nint32 i;\nfor (i=0; i<n;i++) {\ny[i] = 1+A/(1+x[i]/t);\n};"("A"=w346, "t"=w345, "x"=w341, "y"=w341) -> ("y"=w343:dbl[])
              n131 = Bundle("Ramp Pattern"=w341, "y"=w343) -> (w342:cluster{"Ramp Pattern":dbl[], "y":dbl[]})  [unwired: 1 in]
            }
            frame "2D Gaussian + Blinking ACF" {
              n132 = Variant To Data(error in=w361, type=T19 {"Amplitude"=0.0, "Diffusion Time"=0.0, "Blinking Fraction"=0.0, "Blinking Time Constant"=0.0, "RMSE"=0.0, "R^2"=0.0} ("2D Gaussian + Blinking ACF Fit Parameters"), Variant=w362) -> (data=w360:T19, error out=w357:errorcluster)
              n133 = Unbundle By Name(w360) -> ("Amplitude"=w359:dbl, "Diffusion Time"=w358:dbl, "Blinking Fraction"=w352:dbl, "Blinking Time Constant"=w351:dbl)
              n134 = formula code="int32 n = sizeOfDim(x,0);\nint32 i;\nfor (i=0; i<n;i++) {\ny[i] = 1+A/(1+x[i]/t1)*(1-b+b*exp(-x[i]/t2));\n};"("A"=w359, "t1"=w358, "x"=w354, "y"=w354, "b"=w352, "t2"=w351) -> ("y"=w356:dbl[])
              n135 = Bundle("Ramp Pattern"=w354, "y"=w356) -> (w355:cluster{"Ramp Pattern":dbl[], "y":dbl[]})  [unwired: 1 in]
            }
            frame "2D Gaussian + Flow ACF" {
              n136 = Variant To Data(error in=w372, type=T20 {"Amplitude"=0.0, "Diffusion Time"=0.0, "Translation Time"=0.0, "RMSE"=0.0, "R^2"=0.0} ("2D Gaussian + Blinking ACF Fit Parameters"), Variant=w373) -> (data=w371:T20, error out=w368:errorcluster)
              n137 = Unbundle By Name(w371) -> ("Amplitude"=w370:dbl, "Diffusion Time"=w369:dbl, "Translation Time"=w364:dbl)
              n138 = formula code="int32 n = sizeOfDim(x,0);\nint32 i;\nfor (i=0; i<n;i++) {\ny[i] = 1+A/(1+x[i]/t1)*exp(-(x[i]/t2)**2/(1+x[i]/t1));\n};"("A"=w370, "t1"=w369, "x"=w365, "y"=w365, "t2"=w364) -> ("y"=w367:dbl[])
              n139 = Bundle("Ramp Pattern"=w365, "y"=w367) -> (w366:cluster{"Ramp Pattern":dbl[], "y":dbl[]})  [unwired: 1 in]
            }
            frame "3D Gaussian ACF" {
              n140 = Variant To Data(error in=w382, type=T21 {"Amplitude"=0.0, "Diffusion Time"=0.0, "Aspect Ratio"=0.0, "RMSE"=0.0, "R^2"=0.0} ("3D ACF Fit Parameters"), Variant=w384) -> (data=w381:T21, error out=w378:errorcluster)
              n141 = Unbundle By Name(w381) -> ("Aspect Ratio"=w374:dbl, "Amplitude"=w380:dbl, "Diffusion Time"=w379:dbl)
              n142 = formula code="int32 n = sizeOfDim(x,0);\nint32 i;\nfor (i=0; i<n;i++) {\ny[i] = 1+A/(1+x[i]/t)/sqrt(1+x[i]/t/w**2);\n};"("A"=w380, "t"=w379, "x"=w375, "y"=w375, "w"=w374) -> ("y"=w377:dbl[])
              n143 = Bundle("Ramp Pattern"=w375, "y"=w377) -> (w376:cluster{"Ramp Pattern":dbl[], "y":dbl[]})  [unwired: 1 in]
            }
            frame "3D Gaussian + Blinking ACF" {
              n144 = Variant To Data(error in=w396, type=T22 {"Amplitude"=0.0, "Diffusion Time"=0.0, "Aspect Ratio"=0.0, "Blinking Fraction"=0.0, "Blinking Time Constant"=0.0, "RMSE"=0.0, "R^2"=0.0} ("2D Gaussian + Blinking ACF Fit Parameters"), Variant=w397) -> (data=w395:T22, error out=w392:errorcluster)
              n145 = Unbundle By Name(w395) -> ("Amplitude"=w394:dbl, "Diffusion Time"=w393:dbl, "Blinking Fraction"=w388:dbl, "Blinking Time Constant"=w387:dbl, "Aspect Ratio"=w385:dbl)
              n146 = formula code="int32 n = sizeOfDim(x,0);\nint32 i;\nfor (i=0; i<n;i++) {\ny[i] = 1+A/(1+x[i]/t1)/sqrt(1+x[i]/t1/w**2 )*(1-b+b*exp(-x[i]/t2));\n};"("A"=w394, "t1"=w393, "x"=w389, "y"=w389, "b"=w388, "t2"=w387, "w"=w385) -> ("y"=w391:dbl[])
              n147 = Bundle("Ramp Pattern"=w389, "y"=w391) -> (w390:cluster{"Ramp Pattern":dbl[], "y":dbl[]})  [unwired: 1 in]
            }
          }
        }
        frame True {
          n148 = Unbundle By Name(w402) -> ("Show Fit Residuals"=w399:bool, "Residual Type"=w401:T4)
          n149 = Array Size(array=w406) -> (size(s)=w405:i32)
          n150 = Array Size(array=w407) -> (size(s)=w404:i32)
          n151 = Equal?(x=w405, y=w404) -> (x = y?=w403:bool)
          n152 = And(x=w403, y=w399) -> (x .and. y?=w400:bool)
          n153 = case shown="True" w400 {
            tunnel: w409 -> [_ w419]
            tunnel: [_ w418] -> w408
            tunnel: w407 -> [_ w412]
            tunnel: w406 -> [_ w414]
            tunnel: w401 -> [_ w417]
            tunnel: [_ w413] -> w398
            frame False {
            }
            frame True {
              n154 = Compound Arithmetic op=ADD(invert w414, w412) -> (w415:dbl[])
              n155 = case shown="\"Reduced\"" w417 {
                tunnel: [w421 w423 w428] -> w416
                tunnel: w415 -> [w421 w425 w430]
                tunnel: w412 -> [_ w424 w429]
                tunnel: ["Standard Residuals" ("Residual Type") "Normalized Residuals" ("Residual Type") "Reduced Residuals" ("Residual Type")] -> w413
                frame "Standard", Default {
                }
                frame "Normalized" {
                  n156 = Compound Arithmetic op=MULTIPLY(w425, invert w424) -> (w423:dbl[])
                }
                frame "Reduced" {
                  n157 = Square Root(x=w429) -> (sqrt(x)=w427:dbl[])
                  n158 = Compound Arithmetic op=MULTIPLY(w430, invert w427) -> (w428:dbl[])
                }
              }
              n159 = Bundle("X Array in"=w419, w416) -> (w418:cluster{"X Array in":dbl[], dbl[]})  [unwired: 1 in]
            }
          }
          n160 = Bundle("X Array in"=w409, "Best Fit in"=w406) -> (w410:cluster{"X Array in":dbl[], "Best Fit in":dbl[]})  [unwired: 1 in]
        }
      }
    }
    frame Error {
      n161 = Bundle("X Array in"=w433, "Best Fit in"=w432) -> (w431:cluster{"X Array in":dbl[], "Best Fit in":dbl[]})  [unwired: 1 in]
    }
  }
  "Error Out" <- w14
  "Array of Component Plots" <- w3
  "Fitted Plot" <- w2
  "Residual Plot" <- w4
  "Residual Type" <- w5
  n162 = Build Array (concatenate)(w2, w3, w4) -> (→"Array of Plots (Fit, Components, Residuals)":cluster{"X Array in":dbl[], "y":dbl[]}[])
